vi "drawRect.vi"(6 "fill":bool, 7 "input_buffer":u8[](array[numeric]), 8 "h":u8, 9 "w":u8, 10 "y":u8, 11 "x":u8) -> (3 "output_buffer":u8[](array[numeric]) format="%b")   [LabVIEW 2017]
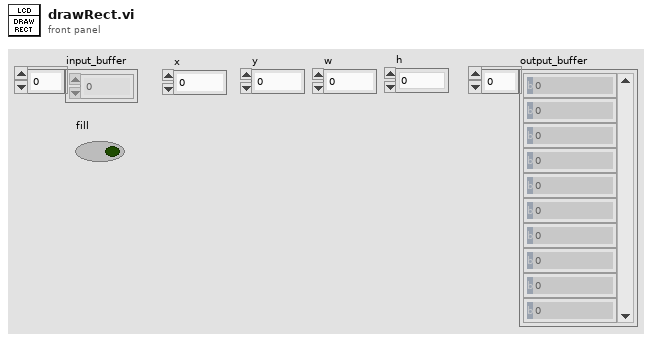
[diagram p1: front panel]
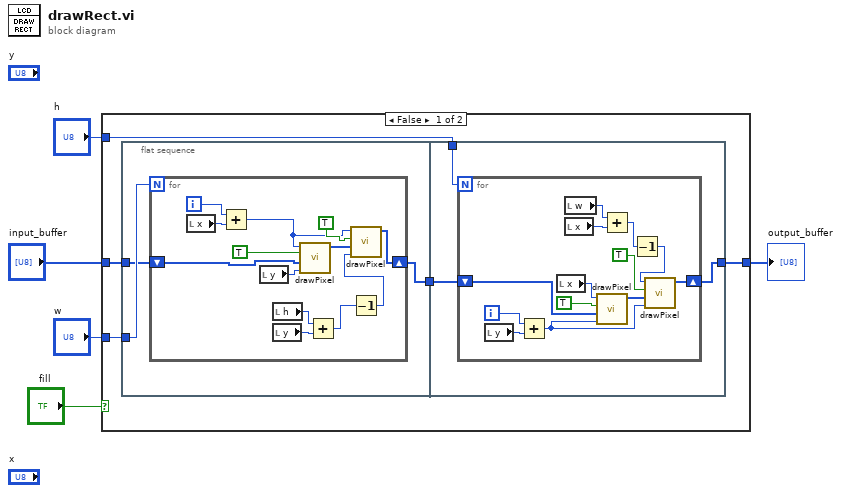
[diagram p0: block diagram]
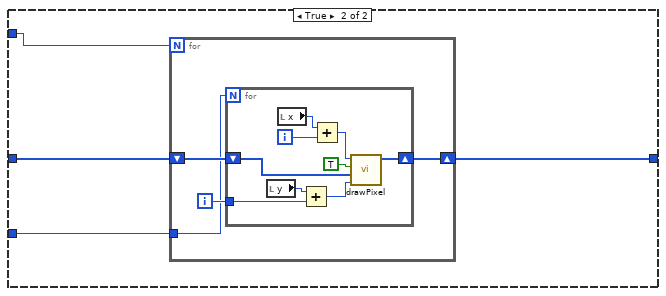
[diagram p2: hidden frame]
diagram:
  n1 = case shown="False" "fill" {
    tunnel: "h" -> [w8 w46]
    tunnel: "w" -> [w10 w45]
    tunnel: "input_buffer" -> [w9 w44]
    tunnel: [w6 w43] -> w2
    frame False {
      n2 = flat-sequence {
        tunnel: w9 -> [w12]
        tunnel: w10 -> [w13]
        tunnel: [w11] -> w7
        tunnel: [w28] -> w6
        tunnel: w8 -> [w29]
        tunnel: w7 -> [w27]
        frame #0 {
          n3 = for {
            N: w13 -> [_]
            shift-right: [w16] -> w11
            shift-left: w12 -> [w23]
            i -> [w22]
            n4 = local read "x"() -> (w25:u8)
            n5 = Add(x=w22, y=w25) -> (x+y=w18:i32)
            n6 = local read "y"() -> (w24:u8)
            n7 = local read "h"() -> (w21:u8)
            n8 = local read "y"() -> (w20:u8)
            n9 = call "drawPixel.vi"("y"=w24, "input_buffer"=w23, "color"=TRUE, "x"=w18) -> ("output_buffer"=w17:u8[])  [unwired: 7 in]
            n10 = Add(x=w21, y=w20) -> (x+y=w15:u8)
            n11 = Decrement(x=w15) -> (x-1=w14:u8)
            n12 = call "drawPixel.vi"("y"=w14, "input_buffer"=w17, "color"=TRUE, "x"=w18) -> ("output_buffer"=w16:u8[])  [unwired: 7 in]
          }
        }
        frame #1 {
          n13 = for {
            N: w29 -> [_]
            shift-right: [w34] -> w28
            shift-left: w27 -> [w39]
            i -> [w41]
            n14 = local read "y"() -> (w40:u8)
            n15 = Add(x=w41, y=w40) -> (x+y=w32:i32)
            n16 = local read "x"() -> (w38:u8)
            n17 = local read "w"() -> (w37:u8)
            n18 = local read "x"() -> (w36:u8)
            n19 = call "drawPixel.vi"("y"=w32, "input_buffer"=w39, "color"=TRUE, "x"=w38) -> ("output_buffer"=w33:u8[])  [unwired: 7 in]
            n20 = Add(x=w37, y=w36) -> (x+y=w31:u8)
            n21 = Decrement(x=w31) -> (x-1=w30:u8)
            n22 = call "drawPixel.vi"("y"=w32, "input_buffer"=w33, "color"=TRUE, "x"=w30) -> ("output_buffer"=w34:u8[])  [unwired: 7 in]
          }
        }
      }
    }
    frame True {
      n23 = for {
        N: w46 -> [_]
        shift-right: [w48] -> w43
        shift-left: w44 -> [w49]
        tunnel: w45 -> [w47]
        i -> [w50]
        n24 = for {
          N: w47 -> [_]
          tunnel: w50 -> [w55]
          shift-right: [w53] -> w48
          shift-left: w49 -> [w54]
          i -> [w57]
          n25 = local read "y"() -> (w51:u8)
          n26 = local read "x"() -> (w52:u8)
          n27 = Add(x=w51, y=w55) -> (x+y=w58:i32)
          n28 = Add(x=w52, y=w57) -> (x+y=w56:i32)
          n29 = call "drawPixel.vi"("y"=w58, "input_buffer"=w54, "color"=TRUE, "x"=w56) -> ("output_buffer"=w53:u8[])  [unwired: 7 in]
        }
      }
    }
  }
  "output_buffer" <- w2
